vi "Power Accuracy Compare and Coerce Stimulus.vi"(6 "Driver Ref (null)":T1, 8 "error in (no error)":errorcluster, 10 "Flat TestSetDef Params":string, 11 "PV Test Parameters":T2={"Stimulus"={"Power Start"=38, "Power Stop"=46, "Frequency Type"=enum."Band Edges", "Frequency Points"=[], "TX 1 Frequency (MHz)"={"Min"=0.0, "Max"=0.0}, "TX 2 Frequency (MHz)"={"Min"=0.0, "Max"=0.0}, "RX Frequency (MHz)"={"Min"=0.0, "Max"=0.0}, "Pad Model Number"="", "Pad Serial Number"="", "Pad Values"=[]}, "Measurement"={"DUT Port"=enum."Port 1", "Direction"=0}, "Display"={"Power"={"Min"=0, "Max"=0}, "Tolerance"={"Min"=0.0, "Max"=0.0}}, "Limit"={"Tolerance"=0.35}, "Calibration"={"Calibrated?"=FALSE}} {"Measurement"."Direction" items=["Reverse", "Forward", "Auxiliary"]}) -> (0 "error out":errorcluster, 3 "Corrected Test Params":T2={"Stimulus"={"Power Start"=38, "Power Stop"=46, "Frequency Type"=enum."Band Edges", "Frequency Points"=[], "TX 1 Frequency (MHz)"={"Min"=0.0, "Max"=0.0}, "TX 2 Frequency (MHz)"={"Min"=0.0, "Max"=0.0}, "RX Frequency (MHz)"={"Min"=0.0, "Max"=0.0}, "Pad Model Number"="", "Pad Serial Number"="", "Pad Values"=[]}, "Measurement"={"DUT Port"=enum."Port 1", "Direction"=0}, "Display"={"Power"={"Min"=0, "Max"=0}, "Tolerance"={"Min"=0.0, "Max"=0.0}}, "Limit"={"Tolerance"=0.35}, "Calibration"={"Calibrated?"=FALSE}} {"Measurement"."Direction" items=["Reverse", "Forward", "Auxiliary"]}, 4 "TestSetDef":T10={"General"={"ID"=0, "Model"="", "Dual Port?"=FALSE, "Options"="", "Options"={"E"=FALSE, "K"=FALSE, "H"=FALSE, "W"=FALSE, "F"=FALSE}, "Cal File"=path ""}, "Receiver"={"Fstart, MHz"=0.0, "Fstop MHz"=0.0, "Fstep MHz"=0.0, "IF, MHz"=0.0}, "RX Band"={"Fstart, MHz"=0.0, "Fstop MHz"=0.0}, "TX 1"={"Fstart, MHz"=0.0, "Fstop MHz"=0.0, "Pmax, dBm"=0.0, "Pstep, dB"=0.0}, "TX 2"={"Fstart, MHz"=0.0, "Fstop MHz"=0.0, "Pmax, dBm"=0.0, "Pstep, dB"=0.0}, "Low-side?"=TRUE})   [LabVIEW 2011]
uses:
  SI.LIB/PIM.LIB/HW IO/Test Set Definition.ctl
  TypeDefs/Power Accuracy Test Parameters.ctl
  TypeDefs/Power Accuracy Stimulus Parameters.ctl
  TypeDefs/Power Accuracy Measurement Parameters.ctl
  SI.LIB/PIM.LIB/HW IO/DUTport.ctl
  SI.LIB/PIM.LIB/HW IO/MeasMode.ctl
  TypeDefs/Power Accuracy Display Parameters.ctl
  TypeDefs/Power Accuracy Limit Parameters.ctl
  TypeDefs/Power Accuracy Calibration State.ctl
  drivers/PIM/PIM Driver Ref.ctl
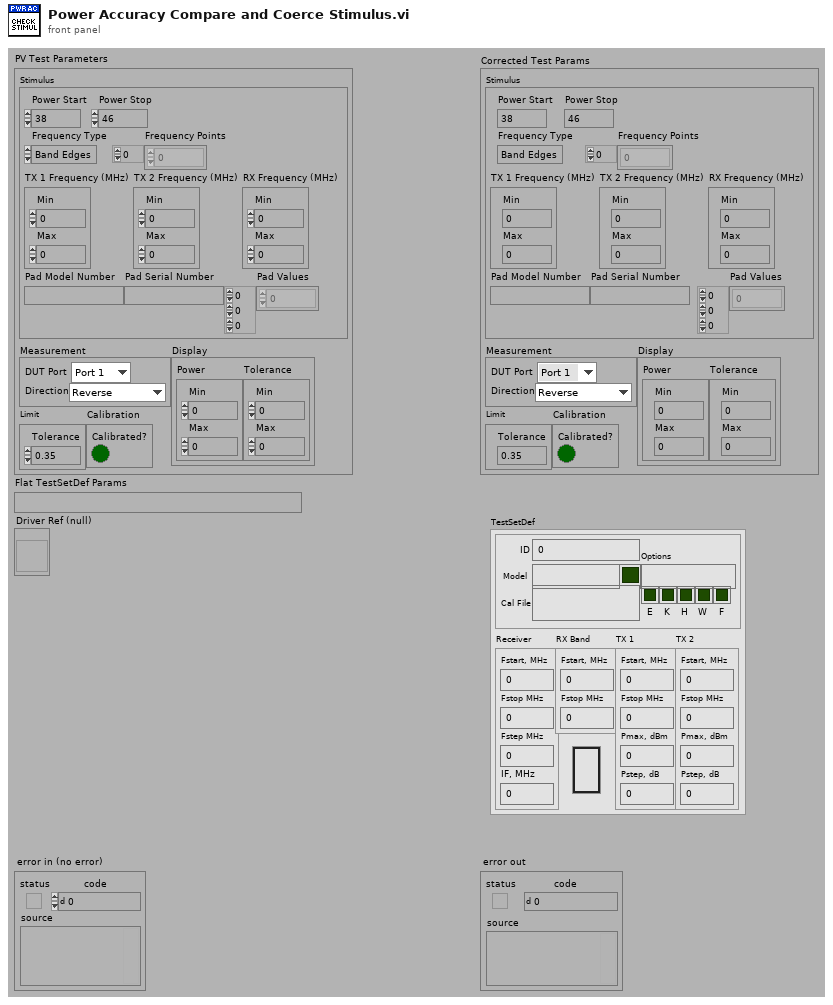
[diagram p1: front panel]
types:
  T1 = typedef "PIM Driver Ref.ctl" = refnum<vi>
  T2 = typedef "Power Accuracy Test Parameters.ctl" = cluster{"Stimulus":T3, "Measurement":T4, "Display":T7, "Limit":T8, "Calibration":T9}
  T3 = typedef "Power Accuracy Stimulus Parameters.ctl" = cluster{"Power Start":i32, "Power Stop":i32, "Frequency Type":enum16{"Band Edges", "Custom"}, "Frequency Points":dbl[], "TX 1 Frequency (MHz)":cluster{"Min":dbl, "Max":dbl}, "TX 2 Frequency (MHz)":cluster{"Min":dbl, "Max":dbl}, "RX Frequency (MHz)":cluster{"Min":dbl, "Max":dbl}, "Pad Model Number":string, "Pad Serial Number":string, "Pad Values":dbl[][][]}
  T4 = typedef "Power Accuracy Measurement Parameters.ctl" = cluster{"DUT Port":T5, "Direction":T6}
  T5 = typedef "DUTport.ctl" = enum16{"Port 1", "Port 2"}
  T6 = typedef "MeasMode.ctl" = u16
  T7 = typedef "Power Accuracy Display Parameters.ctl" = cluster{"Power":cluster{"Min":i32, "Max":i32}, "Tolerance":cluster{"Min":dbl, "Max":dbl}}
  T8 = typedef "Power Accuracy Limit Parameters.ctl" = cluster{"Tolerance":dbl}
  T9 = typedef "Power Accuracy Calibration State.ctl" = cluster{"Calibrated?":bool}
  T10 = typedef "Test Set Definition.ctl" = cluster{"General":cluster{"ID":u32, "Model":string, "Dual Port?":bool, "Options":string, "Options":cluster{"E":bool, "K":bool, "H":bool, "W":bool, "F":bool}, "Cal File":path}, "Receiver":cluster{"Fstart, MHz":dbl, "Fstop MHz":dbl, "Fstep MHz":dbl, "IF, MHz":dbl}, "RX Band":cluster{"Fstart, MHz":dbl, "Fstop MHz":dbl}, "TX 1":cluster{"Fstart, MHz":dbl, "Fstop MHz":dbl, "Pmax, dBm":dbl, "Pstep, dB":dbl}, "TX 2":cluster{"Fstart, MHz":dbl, "Fstop MHz":dbl, "Pmax, dBm":dbl, "Pstep, dB":dbl}, "Low-side?":bool}
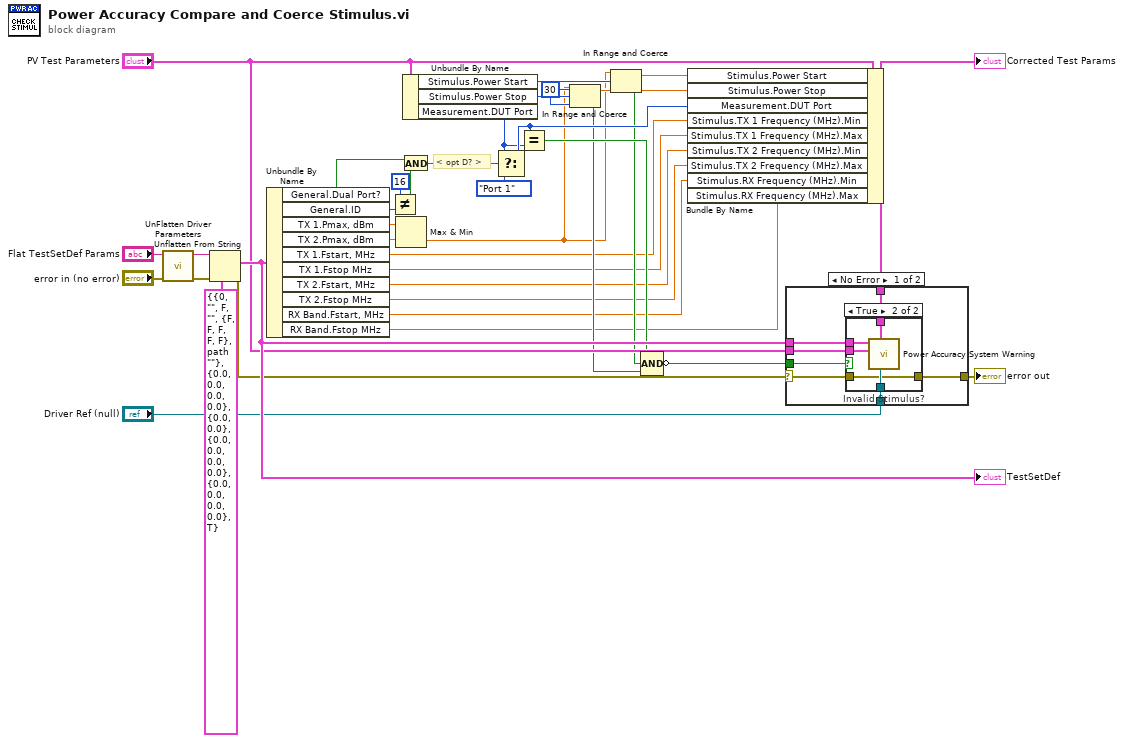
[diagram p0: block diagram]
diagram:
  w2 = 30 ("y")
  # "< opt D? >"
  n1 = call "UnFlatten Driver Parameters.vi"("error in (no error)"="error in (no error)", "Flattened Driver Parameters with Version (\"\")"="Flat TestSetDef Params") -> ("error out"=w33:errorcluster, "Flat Driver Parameters"=w35:string)  [unwired: 4 out]
  n2 = Unflatten From String(type=T10 {"General"={"ID"=0, "Model"="", "Dual Port?"=FALSE, "Options"="", "Options"={"E"=FALSE, "K"=FALSE, "H"=FALSE, "W"=FALSE, "F"=FALSE}, "Cal File"=path ""}, "Receiver"={"Fstart, MHz"=0.0, "Fstop MHz"=0.0, "Fstep MHz"=0.0, "IF, MHz"=0.0}, "RX Band"={"Fstart, MHz"=0.0, "Fstop MHz"=0.0}, "TX 1"={"Fstart, MHz"=0.0, "Fstop MHz"=0.0, "Pmax, dBm"=0.0, "Pstep, dB"=0.0}, "TX 2"={"Fstart, MHz"=0.0, "Fstop MHz"=0.0, "Pmax, dBm"=0.0, "Pstep, dB"=0.0}, "Low-side?"=TRUE} ("Test Set Definition"), binary string=w35, error in (no error)=w33) -> (value=w31:T10, error out=w29:errorcluster)  [unwired: 3 out]
  "TestSetDef" <- w31
  n3 = Unbundle By Name(w31) -> ("General.Dual Port?"=w26:bool, "General.ID"=w22:u32, "TX 1.Pmax, dBm"=w11:dbl, "TX 2.Pmax, dBm"=w10:dbl, "TX 1.Fstart, MHz"=w9:dbl, "TX 1.Fstop MHz"=w8:dbl, "TX 2.Fstart, MHz"=w7:dbl, "TX 2.Fstop MHz"=w6:dbl, "RX Band.Fstart, MHz"=w5:dbl, "RX Band.Fstop MHz"=w4:dbl)
  n4 = Not Equal?(x=16 ("y"), y=w22) -> (x != y?=w27:bool)
  n5 = Max & Min(x=w11, y=w10) -> (min(x,y)=w1:dbl)  [unwired: 1 out]
  n6 = And(x=w26, y=w27) -> (x .and. y?=w24:bool)
  n7 = Unbundle By Name("PV Test Parameters") -> ("Stimulus.Power Start"=w17:i32, "Stimulus.Power Stop"=w13:i32, "Measurement.DUT Port"=w20:T5)
  n8 = Select(t=w20, s=w24, f=DUTport."Port 1" ("Measure.DUT PORT")) -> (s? t:f=w21:T5)
  n9 = Equal?(x=w21, y=w20) -> (x = y?=w19:bool)
  n10 = In Range and Coerce(upper limit=w1, x=w13, lower limit=w2) -> (coerced(x)=w12:dbl, In Range?=w15:bool)
  n11 = In Range and Coerce(upper limit=w1, x=w17, lower limit=w2) -> (coerced(x)=w16:dbl, In Range?=w14:bool)
  n12 = Compound Arithmetic op=AND(w19, w14, w15) -> (invert w32:bool)
  n13 = Bundle By Name(cluster="PV Test Parameters", "Stimulus.Power Start"=w16, "Stimulus.Power Stop"=w12, "Measurement.DUT Port"=w21, "Stimulus.TX 1 Frequency (MHz).Min"=w9, "Stimulus.TX 1 Frequency (MHz).Max"=w8, "Stimulus.TX 2 Frequency (MHz).Min"=w7, "Stimulus.TX 2 Frequency (MHz).Max"=w6, "Stimulus.RX Frequency (MHz).Min"=w5, "Stimulus.RX Frequency (MHz).Max"=w4) -> (w3:T2)
  "Corrected Test Params" <- w3
  n14 = case shown="No Error" w29 {
    selector: w29 -> [w40 w51]
    tunnel: w32 -> [w44 _]
    tunnel: w31 -> [w43 _]
    tunnel: [w42 w51] -> w30
    tunnel: "PV Test Parameters" -> [w41 _]
    tunnel: "Driver Ref (null)" -> [w39 _]
    tunnel: w3 -> [w38 _]
    frame No Error {
      n15 = case "Invalid Stimulus?" shown="True" w44 {
        tunnel: w43 -> [_ w50]
        tunnel: w41 -> [_ w49]
        tunnel: w40 -> [w45 w47]
        tunnel: [w45 w47] -> w42
        tunnel: w39 -> [_ w48]
        tunnel: w38 -> [_ w46]
        frame False {
        }
        frame True {
          n16 = call "Power Accuracy System Warning.vi"("Driver Ref (null)"=w48, "Coerced PV Test Parameters"=w46, "PV Test Parameters"=w49, "TestSetDef"=w50) -> ()  [unwired: 1 in, 7 out]
        }
      }
    }
    frame Error {
      # "If we're in an error state, pass\nthe driver error through to the\nclient machine."
    }
  }
  "error out" <- w30
